vi "Check-Out.vi"(0 "Hotel Management Tool Model in":refnum<class "Hotel Management Tool Model.lvclass">, 5 "Room No":string, 11 "error in (no error)":errorcluster) -> (4 "Hotel Management Tool Model out":refnum<class "Hotel Management Tool Model.lvclass">, 15 "error out":errorcluster)   [LabVIEW 2023, in "Hotel Management Tool Model.lvlib" / "Hotel Management Tool Model.lvclass"]
uses:
  Hotel Management Tool Model.lvclass
  Hotel Management Tool Model.lvclass/Hotel Management Tool Model.ctl
  Central Data Manager/Central Data Manager Messages/Check-Out Msg/Check-Out Msg.lvclass/Check-Out Msg.ctl
  <vilib>/ActorFramework/Message Enqueuer/Message Enqueuer.lvclass/Message Enqueuer.ctl
  <vilib>/ActorFramework/Message Enqueuer/Enqueue.vi
  Central Data Manager/Central Data Manager Messages/Check-Out Msg/Check-Out Msg.lvclass
  C:/Program Files/National Instruments/LabVIEW 2023/vi.lib/ActorFramework/Message/Message.lvclass
  <vilib>/ActorFramework/Message Priority Queue/Priority Enqueue.vi
  <vilib>/ActorFramework/Stop Msg/Stop Msg.lvclass
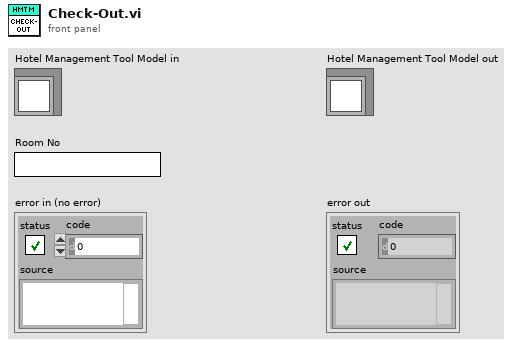
[diagram p1: front panel]
types:
  T1 = map{string, refnum<class "Message Enqueuer.lvclass">}
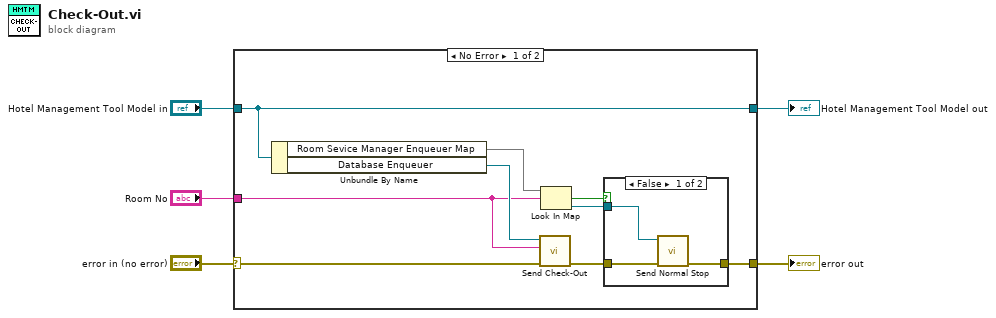
[diagram p0: block diagram]
diagram:
  n1 = case shown="No Error" "error in (no error)" {
    selector: "error in (no error)" -> [w13 w20]
    tunnel: [w8 w20] -> w1
    tunnel: [w14 w19] -> w2
    tunnel: "Hotel Management Tool Model in" -> [w14 w19]
    tunnel: "Room No" -> [w7 _]
    frame No Error {
      n2 = Unbundle By Name(w14) -> ("Room Sevice Manager Enqueuer Map"=w6:T1, "Database Enqueuer"=w12:refnum<class "Message Enqueuer.lvclass">)
      n3 = call "Send Check-Out.vi"("error in (no error)"=w13, "Room No"=w7, "Message Enqueuer"=w12) -> ("error out"=w9:errorcluster)  [unwired: 7 in, 1 out]
      n4 = Look In Map(map=w6, key=w7) -> (key not found?=w10:bool, value=w11:refnum<class "Message Enqueuer.lvclass">)  [unwired: 1 in]
      n5 = case shown="False" w10 {
        tunnel: w9 -> [w17 w18]
        tunnel: [w16 w18] -> w8
        tunnel: w11 -> [w15 _]
        frame False {
          n6 = call <vilib>:"Send Normal Stop.vi"("error in (no error)"=w17, "Message Enqueuer"=w15) -> ("error out"=w16:errorcluster)  [unwired: 9 in]
        }
        frame True {
        }
      }
    }
    frame Error {
    }
  }
  "error out" <- w1
  "Hotel Management Tool Model out" <- w2
